vi "SetTrigger.vi"(8 "error in (no error)":errorcluster, 10 "Trigger":T1, 11 "Photometrics Cam v2 in":refnum<class "Photometrics_CH-250_Cam.lvclass">) -> (0 "error out":errorcluster, 1 "Success":bool, 3 "Photometrics Cam v2 out":refnum<class "Photometrics_CH-250_Cam.lvclass">)   [LabVIEW 2013, in "Photometrics_CH-250_Cam.lvclass"]
uses:
  Photometrics_CH-250_Cam.lvclass
  CameraSessionClass/CS250-CameraHardwareClass.lvclass
  shared/OnOffTypeDef.ctl
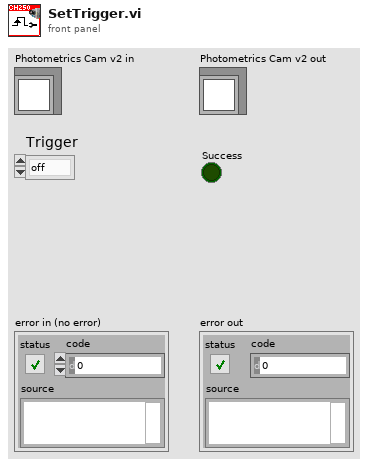
[diagram p1: front panel]
types:
  T1 = typedef "OnOffTypeDef.ctl" = enum16{"off", "on"}
  T2 = typedef "TriggerMode_TypDef.ctl" = enum16{"Timed", "Strobed", "Bulb", "Trigger first", "Flash", "Variable Timed"}
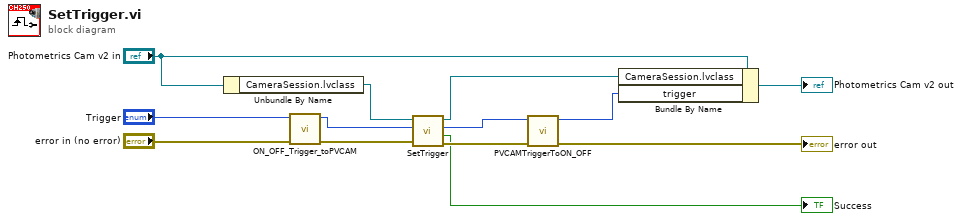
[diagram p0: block diagram]
diagram:
  n1 = Unbundle By Name("Photometrics Cam v2 in") -> ("CameraSession.lvclass"=w7:refnum<class "CS250-CameraHardwareClass.lvclass">)
  n2 = call "ON_OFF_Trigger_toPVCAM.vi"("Trigger"="Trigger") -> ("trigger mode (input)"=w4:T2)  [unwired: 10 in]
  n3 = call-dynamic "SetTrigger.vi"("error in (no error)"="error in (no error)", "TriggerIn"=w4, "CameraSession in"=w7) -> ("error out"=→"error out":errorcluster, "Success"=→"Success":bool, "TriggerOut"=w3:T2, "CameraSession out"=w6:refnum<class "CS250-CameraHardwareClass.lvclass">)  [unwired: 5 in]
  n4 = call "PVCAMTriggerToON_OFF.vi"("TriggerOut"=w3) -> ("y"=w2:T1)  [unwired: 10 in]
  n5 = Bundle By Name(cluster="Photometrics Cam v2 in", "CameraSession.lvclass"=w6, "trigger"=w2) -> (→"Photometrics Cam v2 out":refnum<class "Photometrics_CH-250_Cam.lvclass">)
